vi "SDSU_GBLVariables.vi"() -> ()   [LabVIEW 2016]
panel:
  in  "SDSU_FtimefromHardware":bool
  in  "SDSU_devno":i32
  in  "SDSU_PciStringPath":string
  in  "SDSU_Devices":cluster{"DevNo":u8, "fd":i32}[](array[cluster])
  in  "SDSU_PciInfo":T1 {"RevisionNumber" format="%.0x"; "DeviceID" format="%.0x"; "VendorID" format="%.0x"}
  in  "SDSU_fd":i32
  in  "SDSU_TimingStringPath":string
  in  "SDSU_UtilityStringPath":string
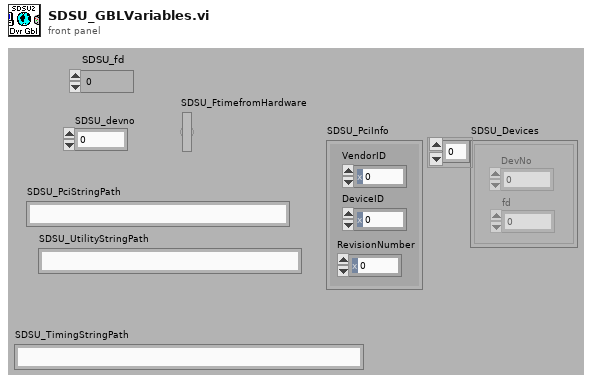
[diagram p1: front panel]
types:
  T1 = cluster{"VendorID":u32, "DeviceID":u32, "RevisionNumber":u32}
diagram:
